vi "action.vi"(0 "NInstrSim_ReadDCMeasurement":refnum<class "NInstrSim_ReadDCMeasurement.lvclass">, 2 "HGF_Visitable":refnum<class "HGF_Visitable.lvclass">, 5 "error in (no error)":errorcluster) -> (14 "dup NInstrSim_ReadDCMeasurement":refnum<class "NInstrSim_ReadDCMeasurement.lvclass">, 16 "dup HGF_Visitable":refnum<class "HGF_Visitable.lvclass">, 19 "error out":errorcluster)   [LabVIEW 2009, in "HB_Device_Examples.lvlib" / "NInstrSim_ReadDCMeasurement.lvclass"]
doc: "This is a dynamic dispatch VI that is called from Visitor.visit(). It will call member VIs of Visitable to perform the requested action which means: calling public methods of Visitable child class.\n\n<B>Hint:</B> This method is abstract and need to be implemented by child classes."
uses:
  NInstrSim_ReadDCMeasurement.lvclass
  lib.lib/HGF_LVC/HGF_BaseClasses/HGF_Visitable/HGF_Visitable.lvclass
  NInstrSim.lvclass
  NInstrSim_ReadDCMeasurement.lvclass/NInstrSim_ReadDCMeasurement.ctl
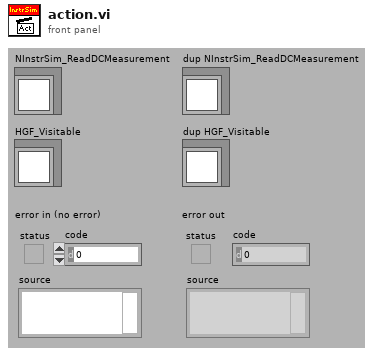
[diagram p1: front panel]
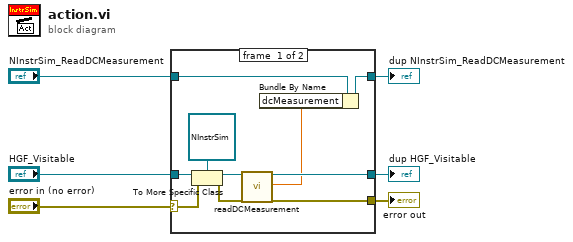
[diagram p0: block diagram]
diagram:
  n1 = case shown="No Error" "error in (no error)" {
    selector: "error in (no error)" -> [w14 w17]
    tunnel: "NInstrSim_ReadDCMeasurement" -> [w9 w19]
    tunnel: "HGF_Visitable" -> [w16 w18]
    tunnel: [w12 w18] -> w4
    tunnel: [w10 w17] -> w3
    tunnel: [w8 w19] -> w1
    frame #0 {
      n2 = To More Specific Class(target class=refnum<class "NInstrSim.lvclass"> refnum ("HB_HGF_Test.lvlib:NInstrSim.lvclass"), reference=w16, error in=w14) -> (specific class reference=w13:refnum<class "NInstrSim.lvclass">, error out=w11:errorcluster)
      n3 = call "readDCMeasurement.vi"("NInstrSim"=w13, "error in (no error)"=w11) -> ("dup NInstrSim"=w12:refnum<class "NInstrSim.lvclass">, "DC Measurement"=w7:dbl, "error out"=w10:errorcluster)  [unwired: 15 out]
      n4 = Bundle By Name(cluster=w9, "dcMeasurement"=w7) -> (w8:refnum<class "NInstrSim_ReadDCMeasurement.lvclass">)
    }
    frame #1 {
    }
  }
  "error out" <- w3
  "dup NInstrSim_ReadDCMeasurement" <- w1
  "dup HGF_Visitable" <- w4
